vi "changeState.vi"(8 "error in (no error)":errorcluster, 10 "State:":T1=enum."FaultState", 11 "Model in":refnum<class "Model.lvclass">) -> (0 "error out":errorcluster, 3 "Model out":refnum<class "Model.lvclass">)   [LabVIEW 2013, in "Model.lvclass"]
uses:
  Model.lvclass
  Typedefs/StateSelector.ctl
  Model.lvclass/Model.ctl
  ApplicationElements/Log/TestDataLog/TestDataLog.lvclass/TestDataLog.ctl
  UserEvents/UserEvents.lvclass/UserEvents.ctl
  UserEvents/UserEvents.lvclass
  ApplicationElements/Log/TestDataLog/TestDataLog.lvclass
  Typedefs/ILCBTTypedefs.lvlib
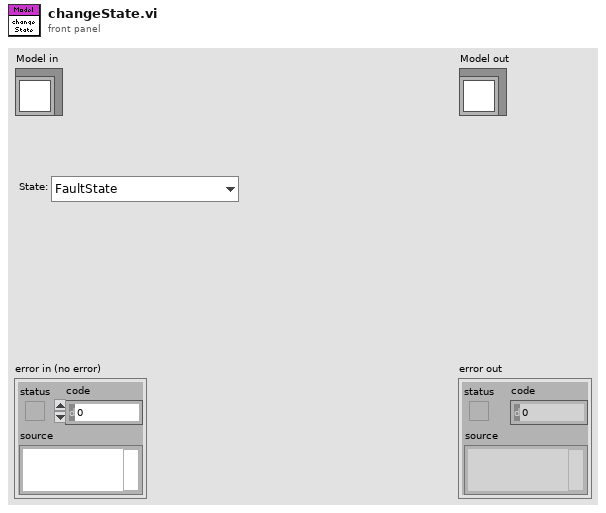
[diagram p1: front panel]
types:
  T1 = typedef "ILCBTTypedefs.lvlib/StateSelector.ctl" = enum16{"EnabledState", "FaultState", "OffState", "StandbyState"}
  T2 = typedef "ILCBTTypedefs.lvlib/PubDataEvents.ctl" = cluster{"State":refnum<user-event>, "ErrorCode":refnum<user-event>, "OutputData":refnum<user-event>, "LogPath":refnum<user-event>}
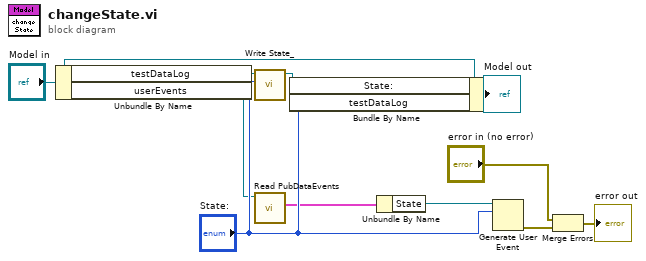
[diagram p0: block diagram]
diagram:
  n1 = Unbundle By Name("Model in") -> ("testDataLog"=w6:refnum<class "TestDataLog.lvclass">, "userEvents"=w3:refnum<class "UserEvents.lvclass">)
  n2 = call "Write State_.vi"("State:"="State:", "TestDataLog in"=w6) -> ("TestDataLog out"=w4:refnum<class "TestDataLog.lvclass">)  [unwired: 9 in]
  n3 = call "Read PubDataEvents.vi"("UserEvents in"=w3) -> ("PubDataEvents"=w2:T2)  [unwired: 9 in, 1 out]
  n4 = Bundle By Name(cluster="Model in", "State:"="State:", "testDataLog"=w4) -> (→"Model out":refnum<class "Model.lvclass">)
  n5 = Unbundle By Name(w2) -> ("State"=w1:refnum<user-event>)
  n6 = Generate User Event(user event=w1, event data cluster="State:") -> (error out=w8:errorcluster)  [unwired: 2 in, 1 out]
  n7 = Merge Errors("error in (no error)", w8) -> (→"error out":errorcluster)
